vi "1.vi"() -> ()   [LabVIEW 2023]
uses:
  <vilib>/Platform/TimedLoop/XDataNode/timing_clust.ctl
  <vilib>/Platform/TimedLoop/XDataNode/nitl_modes.ctl
  <vilib>/Platform/TimedLoop/XDataNode/wakeup.ctl
  <vilib>/platform/TimedLoop/XDataNode/XDataNode.xnode
  <vilib>/Platform/TimedLoop/XDataNode/XDNodeRunTimeDep.lvlib
panel:
  out "consignapwm":u32
  in  "consignapwm":u32
  out "medida sensor":cluster{"number 2":i32, "number 2":i32}(graph)
  out "consigna":i32
  out "indice 2":i32
  in  "Dial":dbl(knob) scale=0.0..6000.0
  out "String":string
  out "sensor":i32
  out "indice 1":i32
  in  "Mandar":string
  out "Recibido":string
  in  "Puerto":refnum<visa-resource-name>
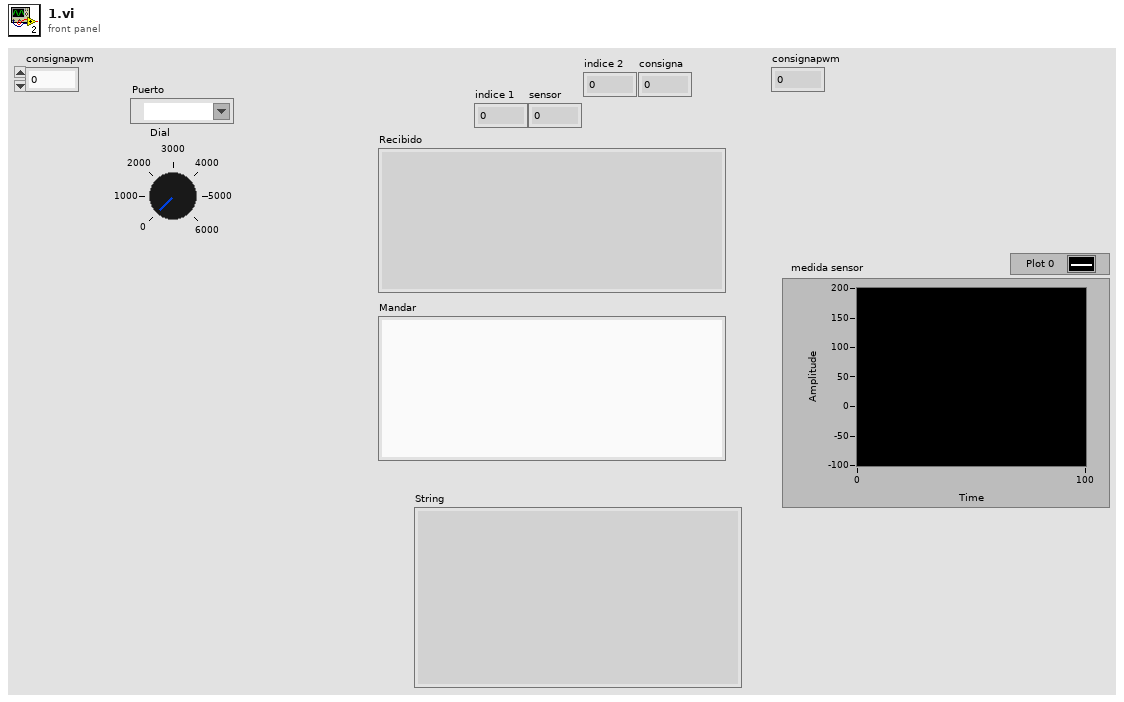
[diagram p1: front panel]
types:
  T1 = typedef "XDNodeRunTimeDep.lvlib/timing_clust.ctl" = cluster{"Expected End [f-1]":u64, "Actual End [f-1]":u64, "Finished Late? [f-1]":bool, "Expected End [i-1]":u64, "Actual End [i-1]":u64, "Finished Late? [i-1]":bool, "Expected Start [i]":u64, "Actual Start [i]":u64, "Expected Start [f]":u64, "Actual Start [f]":u64, "Source Name":string, "Structure Name":string, "Period":i64, "Deadline":i64, "Offset":i64, "Start":i64, "Priority":i32, "Timeout":i32, "Mode":T2, "Wakeup Reason":T3, "Error":errorcluster, "Source Type":string, "Secondary Source Type":string, "Global End Time":u64, "Global Start Time":u64, "Frame Duration":u64, "Iteration Duration":u64, "Assigned CPU":i32, "I/O Scan Engine Mode":u32}
  T2 = typedef "XDNodeRunTimeDep.lvlib/nitl_modes.ctl" = enum32{"No Change", "Process missed periods, maintain original phase", "Discard missed periods, maintain original phase", "Process missed periods, ignore original phase", "Discard missed periods, ignore original phase"}
  T3 = typedef "XDNodeRunTimeDep.lvlib/wakeup.ctl" = enum32{"Normal", "Aborted", "Asynchronous wakeup", "Timing source error", "Timed loop error", "Timeout"}
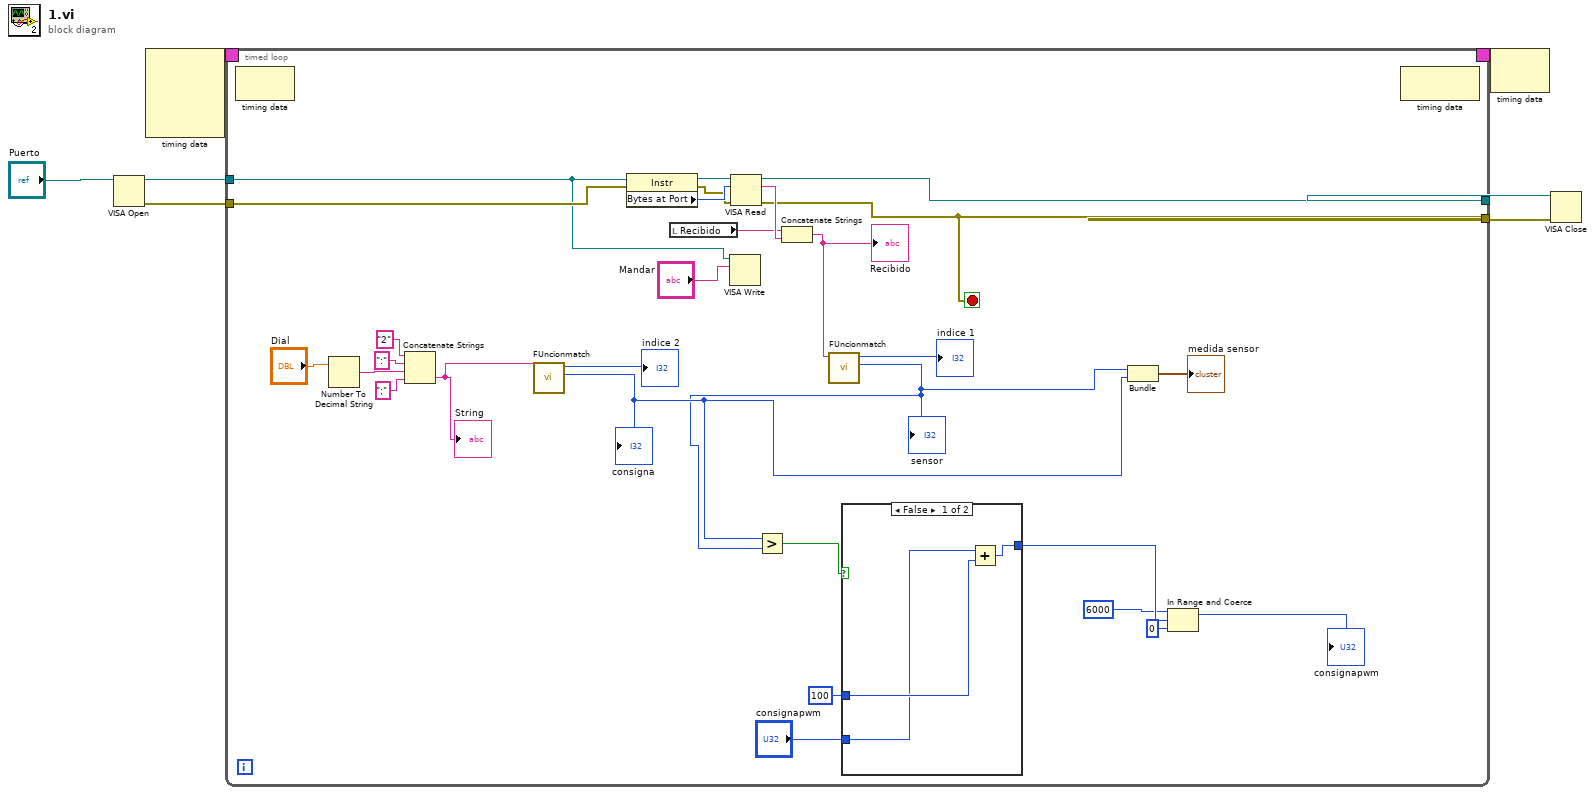
[diagram p0: block diagram]
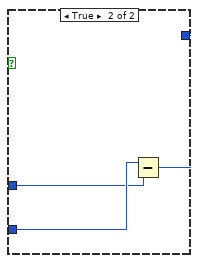
[diagram p2: hidden frame]
diagram:
  n1 = VISA Open(VISA resource name="Puerto") -> (VISA resource name=w4:refnum<visa-resource-name>, error out=w3:errorcluster)  [unwired: 4 in]
  n2 = node-c288() -> (w6:T1)  [unwired: 4 in]
  n3 = timed-loop {
    timing: w6 -> [_]
    timing-out: [_] -> w5
    tunnel: w4 -> [w29]
    tunnel: w3 -> [w36]
    tunnel: [w32] -> w2
    tunnel: [w27] -> w1
    stop <- w27 stop-if-true
    n4 = node-c288() -> ()  [unwired: 1 in, 1 out]
    n5 = Number To Decimal String(number="Dial") -> (decimal integer string=w24:string)  [unwired: 1 in]
    n6 = Concatenate Strings("2" ("string"), ":" ("string"), w24, ";" ("string")) -> (w18:string)
    "String" <- w18
    n7 = call "FUncionmatch.vi"("Entrada"=w18) -> ("number 2"=w16:i32, "number"=→"indice 2":i32)  [unwired: 8 in, 1 out]
    "consigna" <- w16
    n8 = property class="Instr"(reference=w29, error in=w36) -> (reference out=w33:refnum<visa-resource-name>, error out=w34:errorcluster, "Bytes at Port"=w35:u32)
    n9 = local read "Recibido"() -> (w30:string)
    n10 = VISA Write(VISA resource name=w29, write buffer="Mandar") -> ()  [unwired: 1 in, 3 out]
    n11 = VISA Read(VISA resource name=w33, byte count=w35, error in (no error)=w34) -> (VISA resource name out=w32:refnum<visa-resource-name>, read buffer=w31:string, error out=w27:errorcluster)  [unwired: 1 out]
    n12 = Concatenate Strings(w30, w31) -> (w26:string)
    "Recibido" <- w26
    n13 = call "FUncionmatch.vi"("Entrada"=w26) -> ("number 2"=w15:i32, "number"=→"indice 1":i32)  [unwired: 8 in, 1 out]
    "sensor" <- w15
    n14 = Greater?(x=w16, y=w15) -> (0:w14:bool)
    n15 = case shown="False" w14 {
      tunnel: [w39 w40] -> w11
      tunnel: "consignapwm" -> [w37 w42]
      tunnel: u32 100 ("cte") -> [w38 w41]
      frame False {
        n16 = Add(x=w37, y=w38) -> (x+y=w39:u32)
      }
      frame True {
        n17 = Subtract(x=w42, y=w41) -> (x-y=w40:u32)
      }
    }
    n18 = Bundle("number 2"=w15, "number 2"=w16) -> (→"medida sensor":cluster{"number 2":i32, "number 2":i32})  [unwired: 1 in]
    n19 = In Range and Coerce(upper limit=u32 6000, x=w11, lower limit=u32 0) -> (coerced(x)=→"consignapwm":u32)  [unwired: 1 out]
    n20 = node-c288() -> ()  [unwired: 1 in, 1 out]
  }
  n21 = node-c288(w5) -> ()  [unwired: 1 out]
  n22 = VISA Close(VISA resource name=w2, error in (no error)=w1) -> ()  [unwired: 1 out]
